vi "Solar Position Calculator - Meeus.vi"(11 "Observer's Latitude":dbl=39.977726 format="%#_8g", 13 "Observer's Longitude":dbl=105.274512 format="%#_9g") -> (9 "LST [Deg]":ext=222.68484852563896581 format="%_6g", 14 "Apparent Solar RA (deg)":dbl=243.2050632762713 format="%.6f", 15 "Apparent Solar Dec (deg)":dbl=-21.152223700920082 format="%.6f", 16 "Solar Altitude":dbl=25.94308858867875 format="%#_10g", 17 "Solar Azimuth":dbl=158.68124009009193 format="%#_10g", 18 "System Time and Date":T2={"current local time"=timestamp(3531489986.983003 s since 1904-01-01), "Julian Date"=2457354.2267004647, "LST [hh:mm:ss]"="14:50:44.4"} {"Julian Date" format="%_12f"}, 19 "Solar Position":T1={"Azimuth"=158.68124009009193, "Altitude wrt Horizon"=25.94308858867875, "Apparent RA (h:m:s)"="16:12:49.2", "Apparent Declination [dms]"="-21:9:8.005"} {"Altitude wrt Horizon" format="%.3f"; "Azimuth" format="%.3f"})   [LabVIEW 2015]
doc: "Solar Coordinates with High Accuracy, \"Astronomical Algorithms\" by Jean Meeus, pg. 166\n\nUsing data from Appendix III, (for the earth), calculate the earth's heliocentric longitude \"L\" and latitutde \"B\", and the radius vector \"R\" for a given instant as explained in chapter 32\n\nTime 'tau' is measured from JDE 2451545.0 in Julian mellenia (365250 days), NOT in centures and that the final values for \"L\" and \"B\" are in radians.\n\nChapter 32: \"Positions of the Planets\" \n The osculating orbit (using long series of periodic terms) is the \"instantaneous\" orbit with the following values:\n\n a = semi-major axis of the orbit\n lambda = mean longitude of the planet\n h = e sin (pi)\n k = e cos (pi)\n p = sin (1/2 i) sin (Omega)\n q = sin(1/2 i) cos (Omega)\n\n where 'e' is the orbital eccentricity\n 'pi' is the longitude of the perihelion\n 'i' is the inclination and\n 'Omega' is the longitude of the ascending node"
panel:
  out "Sun's Apparent Longitude\nCorrected for Aberration":dbl=245.13904264450866 format="%#_8g"
  out "Julian centuries (T)":ext=0.15904795894496178561 format="%_10g"
  out "Sun's Apparent Longitude":string="245:8:18.627"
  out "Sun's Apparent Longitude\nCorrected for Nutation and Aberration":dbl=245.13850753497218 format="%_8g"
  out "Equation \n25.10":dbl=-20.76572876500679
  out "Laskar True Obliquity [Deg]":dbl=23.43451957510621 format="%#_10g"
  out "Ecliptic Latitude [dms]":string="359:59:59.442"
  out "Ecliptic Latitude (FK)":dbl=359.9998448896821
  out "FK5 Longitude":dbl=245.14481090249893 format="%#_9g"
  out "Geocentric Solar Latitude":string="359:59:59.398"
  out "Deg:Min:Sec":string="245:8:41.319"
  out "series sum for d(epsilon) [\"]":dbl=-9.732610111354601 format="%#_4g"
  out "series sum for d(psi) [\"]":dbl=-1.9263943312994156 format="%#_5g"
  out "Laskar True Obliquity [DMS]":string="23:26:4.270"
  out "Latitude Correction \nfor Change from VSOP to FK5 System\n[arc seconds]":dbl=0.043620587030384496 format="%#_2g"
  in  "Longitude Correction\nfor Change from VSOP to FK6 System\n[deg] see page 166-169 of Meeus":dbl=-2.5e-05 format="%_4f"
  out "L' [FK5 System]":dbl=244.9226380620143 format="%#_5g"
  out "T":dbl=0.15904795894496176 format="%#_10g"
  out "Geocentric Latitude of the Sun [deg]":dbl=359.99983277285236 format="%#_4g"
  out "Geocentric Longitude of the Sun":dbl=245.14483590249893 format="%#_9g"
  out "B [deg]":dbl=0.00016722714764220623 format="%#_4g"
  out "L [0-360]":dbl=65.14483590249893 format="%#_8g"
  out "L [deg]":dbl=5825.144835902499 format="%#_10g"
  out "R [AU]":dbl=0.9867123004384141 format="%#_8g"
  out "B [rad]":dbl=2.918664325075171e-06 format="%#_3f"
  out "L [rad]":dbl=101.66795679204338 format="%#_10g"
  out "Julian Millenia (tau)":dbl=0.015904795894496178 format="%#_10g"
  in  "L0 - Earthm [64 terms]":dbl[][](array[numeric])=[[175347046.0, 0.0, 0.0], [3341656.0, 4.6692568, 6283.07585], [34894.0, 4.6261, 12566.1517], [3497.0, 2.7441, 5753.3849], [3418.0, 2.8289, 3.5231], [3136.0, 3.6277, 77713.7715], [2676.0, 4.4181, 7860.4194], [2343.0, 6.1352, 3930.2097], [1324.0, 0.7425, 11506.7698], [1273.0, 2.0371, 529.691], [1199.0, 1.1096, 1577.3435], [990.0, 5.233, 5884.927], [902.0, 2.045, 26.298], [857.0, 3.508, 398.149], [780.0, 1.179, 5223.694], [753.0, 2.533, 5507.553], [505.0, 4.583, 18849.228], [492.0, 4.205, 775.523], [357.0, 2.92, 0.067], [317.0, 5.849, 11790.629], [284.0, 1.899, 796.298], [271.0, 0.315, 10977.079], [243.0, 0.345, 5486.778], [206.0, 4.806, 2544.314], [205.0, 1.869, 5573.143], [202.0, 2.458, 6069.777], [156.0, 0.833, 213.299], [132.0, 3.411, 2942.463], [126.0, 1.083, 20.775], [115.0, 0.645, 0.98], [103.0, 0.636, 4694.003], [102.0, 0.976, 15720.839], [102.0, 4.267, 7.114], [99.0, 6.21, 2146.17], [98.0, 0.68, 155.42], [86.0, 5.98, 161000.69], [85.0, 1.3, 6275.96], [85.0, 3.67, 71430.7], [80.0, 1.81, 17260.15], [79.0, 3.04, 12036.46], [75.0, 1.76, 5088.63], [74.0, 3.5, 3154.69], [74.0, 4.68, 801.82], [70.0, 0.83, 9437.76], [62.0, 3.98, 8827.39], [61.0, 1.82, 7084.9], [57.0, 2.78, 6286.6], [56.0, 4.39, 14143.5], [56.0, 3.47, 6279.55], [52.0, 0.19, 12139.55], [52.0, 1.33, 1748.02], [51.0, 0.28, 5856.48], [49.0, 0.49, 1194.45], [41.0, 5.37, 8429.24], [41.0, 2.4, 19651.05], [39.0, 6.17, 10447.39], [37.0, 6.04, 10213.29], [37.0, 2.57, 1059.38], [36.0, 1.71, 2352.87], [36.0, 1.78, 6812.77], [33.0, 0.59, 17789.85], [30.0, 0.44, 83996.85], [30.0, 2.74, 1349.87], [25.0, 3.16, 4690.48]] format="%#_12g"
  in  "L1 - Earth [34 terms]":dbl[][](array[numeric])=[[628331966747.0, 0.0, 0.0], [206059.0, 2.678235, 6283.07585], [4303.0, 2.678235, 12566.1517], [425.0, 1.59, 3.523], [119.0, 5.796, 26.298], [109.0, 2.966, 1577.344], [93.0, 2.59, 18849.23], [72.0, 1.14, 529.69], [68.0, 1.87, 398.15], [67.0, 4.41, 5507.55], [59.0, 2.89, 5223.69], [56.0, 2.17, 155.42], [45.0, 0.4, 796.3], [36.0, 0.47, 775.52], [29.0, 2.65, 7.11], [21.0, 5.34, 0.98], [19.0, 1.85, 5486.78], [19.0, 4.97, 213.3], [17.0, 2.99, 6275.96], [16.0, 0.03, 2544.31], [16.0, 1.43, 2146.17], [15.0, 1.21, 10977.08], [12.0, 2.83, 1748.02], [12.0, 3.26, 5088.63], [12.0, 5.27, 1194.45], [12.0, 2.08, 4694.0], [11.0, 0.77, 553.57], [10.0, 1.3, 6286.6], [10.0, 4.24, 1349.87], [9.0, 2.7, 242.73], [9.0, 5.64, 951.72], [8.0, 5.3, 2352.87], [6.0, 2.65, 9437.76], [6.0, 4.67, 4690.48]] format="%#_12g"
  in  "L2 - Earth [20 terms]":dbl[][](array[numeric])=[[52919.0, 0.0, 0.0], [8720.0, 1.0721, 6283.0758], [309.0, 0.867, 12566.152], [27.0, 0.05, 3.52], [16.0, 5.19, 26.3], [16.0, 3.68, 155.42], [10.0, 0.76, 18849.23], [9.0, 2.06, 77713.77], [7.0, 0.83, 775.52], [5.0, 4.66, 1577.34], [4.0, 1.03, 7.11], [4.0, 3.44, 5573.14], [3.0, 5.14, 796.3], [3.0, 6.05, 5507.55], [3.0, 1.19, 242.73], [3.0, 6.12, 529.69], [3.0, 0.31, 398.15], [3.0, 2.28, 553.57], [2.0, 4.38, 5223.69], [2.0, 3.75, 0.98]] format="%#_12g"
  in  "L3 - Earth [7 terms]":dbl[][](array[numeric])=[[289.0, 5.844, 6283.076], [35.0, 0.0, 0.0], [17.0, 5.49, 12566.15], [3.0, 5.2, 155.42], [1.0, 4.72, 3.52], [1.0, 5.3, 18849.23], [1.0, 5.97, 242.73]] format="%#_12g"
  in  "L4 - Earth [3 terms]":dbl[][](array[numeric])=[[114.0, 3.142, 0.0], [8.0, 4.13, 6283.08], [1.0, 3.84, 12566.15]] format="%#_12g"
  in  "L5 - Earth [1 term]":dbl[][](array[numeric])=[[1.0, 3.14, 0.0]] format="%#_12g"
  in  "R0 - Earth [40 terms]":dbl[][](array[numeric])=[[100013989.0, 0.0, 0.0], [1670700.0, 3.0984635, 6283.07585], [13956.0, 3.05525, 12566.1517], [3084.0, 5.1985, 77713.7715], [1628.0, 1.1739, 5753.5849], [1576.0, 2.8469, 7860.4194], [925.0, 5.453, 11506.77], [542.0, 4.564, 3930.21], [472.0, 3.661, 5884.927], [346.0, 0.964, 5507.553], [329.0, 5.9, 5223.694], [307.0, 0.299, 5573.143], [243.0, 4.273, 11790.629], [212.0, 5.847, 1577.344], [186.0, 5.022, 10977.079], [175.0, 3.012, 18849.228], [110.0, 5.055, 5486.778], [98.0, 0.89, 6069.78], [86.0, 5.69, 15720.84], [86.0, 1.27, 161000.69], [65.0, 0.27, 17260.15], [63.0, 0.92, 529.69], [57.0, 2.01, 83996.85], [56.0, 5.24, 71430.7], [49.0, 3.25, 2544.31], [47.0, 2.58, 775.52], [45.0, 5.54, 9437.76], [43.0, 6.01, 6275.96], [39.0, 5.36, 4694.0], [38.0, 2.39, 8827.39], [37.0, 0.83, 19651.05], [37.0, 4.9, 12139.55], [36.0, 1.67, 12036.46], [35.0, 1.84, 2942.46], [33.0, 0.24, 7084.9], [32.0, 0.18, 5088.63], [32.0, 1.78, 398.15], [28.0, 1.21, 6286.6], [28.0, 1.9, 6279.55], [26.0, 4.59, 10447.39]] format="%#_12g"
  in  "R1 - Earth [10 terms]":dbl[][](array[numeric])=[[103019.0, 1.10749, 6283.07585], [1721.0, 1.0644, 12566.1517], [702.0, 3.142, 0.0], [32.0, 1.02, 18849.23], [31.0, 2.84, 5507.55], [25.0, 1.32, 5223.69], [18.0, 1.42, 1577.34], [10.0, 5.91, 10977.08], [9.0, 1.42, 6275.96], [9.0, 0.27, 5486.78]] format="%#_12g"
  in  "R2 - Earth [6-terms]":dbl[][](array[numeric])=[[4359.0, 5.7846, 6283.07585], [124.0, 5.579, 12566.152], [12.0, 3.14, 0.0], [9.0, 3.63, 77713.77], [6.0, 1.87, 5573.14], [3.0, 5.47, 18849.23]] format="%#_12g"
  in  "R4 - Earth [1-term]":dbl[][](array[numeric])=[[4.0, 2.56, 6283.08]] format="%#_12g"
  in  "R3 - Earth [2-terms]":dbl[][](array[numeric])=[[145.0, 4.273, 6283.076], [7.0, 3.92, 12566.15]] format="%#_12g"
  in  "B1 - Earth [2 terms]":dbl[][](array[numeric])=[[9.0, 3.9, 5507.55], [6.0, 1.73, 5223.69]] format="%#_12g"
  in  "B0 - Earth [5 terms]":dbl[][](array[numeric])=[[280.0, 3.199, 84334.662], [102.0, 5.422, 5507.553], [80.0, 3.88, 5223.69], [44.0, 3.7, 2352.87], [32.0, 4.0, 1577.34]] format="%#_12g"
  # "These are the heliocentric longitude \"L\", latitude \"B\" \nreferred to the mean dynamical ecliptic."
  # "These are the geocentric \"L\" and \"B\"\nof the SUN, still referred to the mean\ndynamical ecliptic"
  # "The sun's longitude thus far is the true \n\"geometric\" longitude.  To obtain the apparent \nlongitude, lambda, the effects of nutation \nand abberation should be taken into account.\n\nNutation is calculated by means from Chapter 22."
  # "Converting to FK5 System"
  # "`"
  # "These corrections may be neglected\nwhen using the abridged VSOP version\nfrom Appendix III of Meeus"
  # "Using latlong.net, I determined the position of the Mesa Lab Dome to be\n39.977726, -105.274512"
  # "NOAA Solar Position Calculator \nNew: http://www.esrl.noaa.gov/gmd/grad/solcalc/\nOld http://www.srrb.noaa.gov/highlights/sunrise/azel.html\n\nDefault Values for Mesa Lab Spar\n39.977727 degrees latitude\n-105.274512 degrees (west of prime meridian)\n\nJPL Horizons Calculator \nhttp://ssd.jpl.nasa.gov/horizons.cgi\n\nEphemeris Type: Observer\nTarget Body: Sun [Sol] \nObserver Location: user defined (105N15'39.6\"E, 39:59:27.6\" N, 6000 ft)\nTime Span: user defined Start: 2015-03-24, Stop 2015-03-25, Step - 1min)\nTable Settings: Qantities 2,13,36, CSV format = YES, angle format can be either DEG or HMS\nDisplay/Output: default (can be sent to a text file)"
  # "Ecliptic Solar Coordinates"
  # "Horizon Solar Coordinates"
  # "Apparent Equatorial Solar Coordinates"
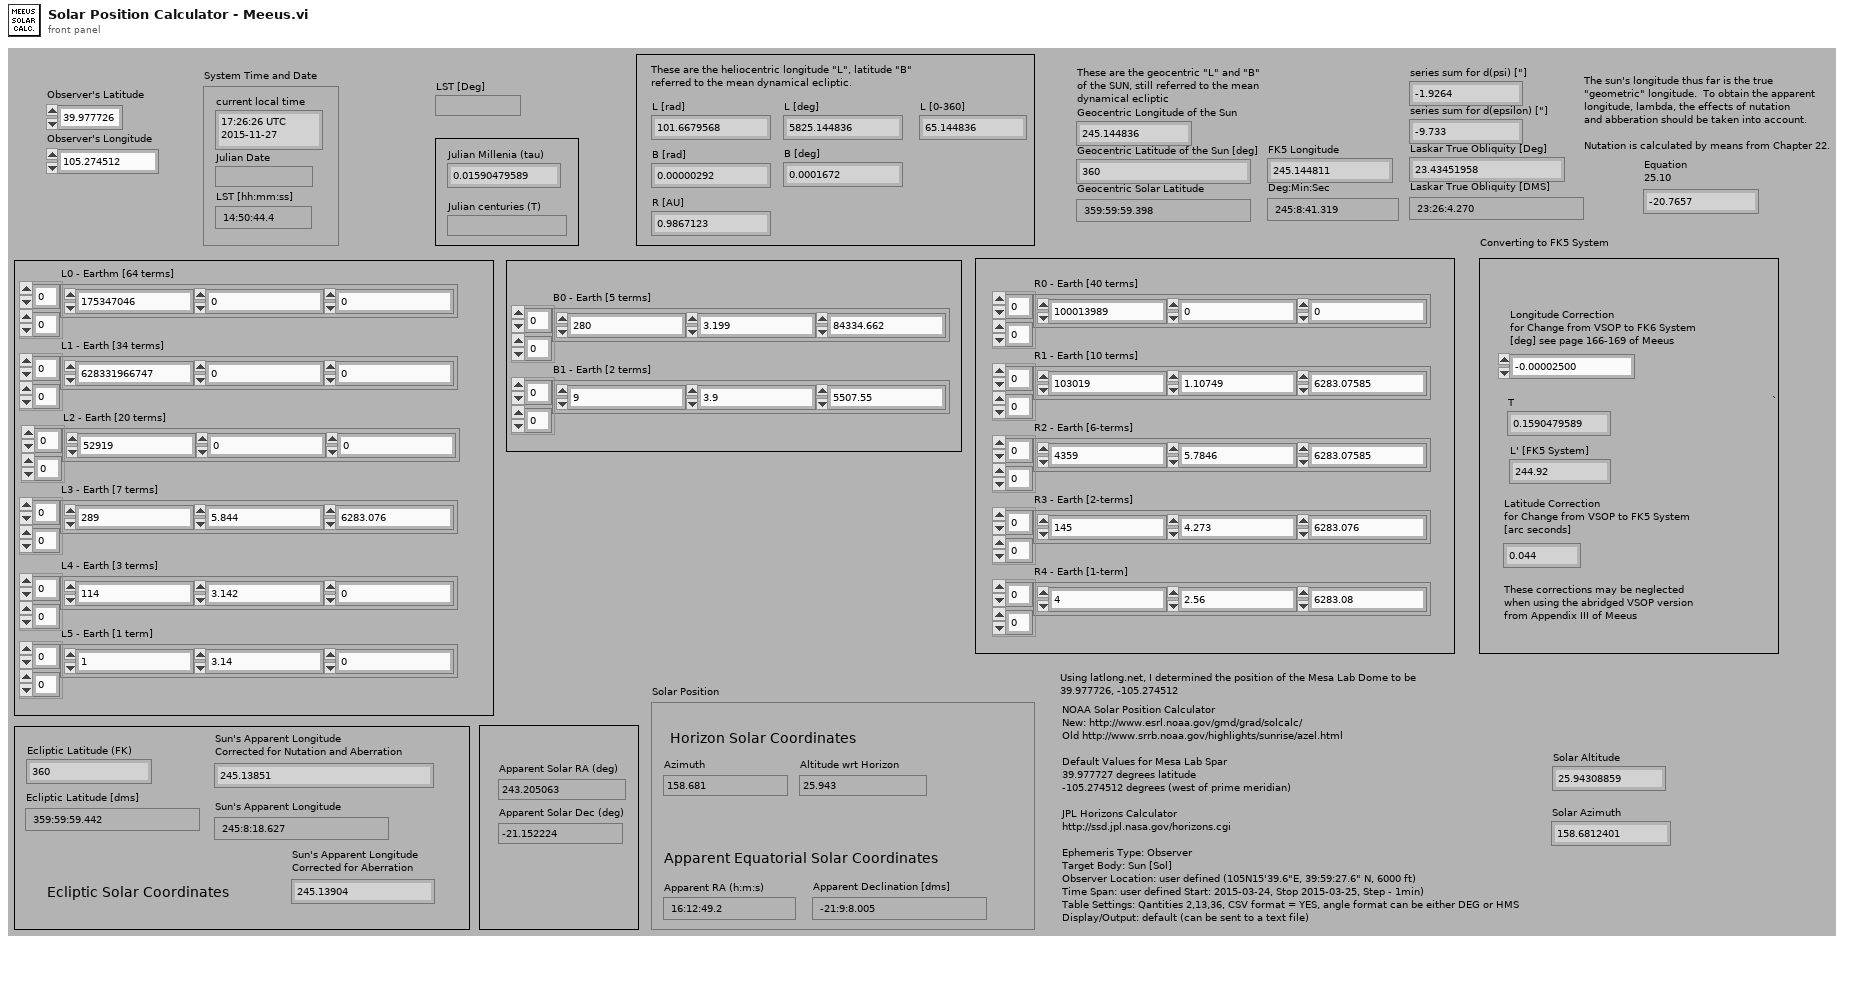
[diagram p1: front panel]
types:
  T1 = cluster{"Azimuth":dbl, "Altitude wrt Horizon":dbl, "Apparent RA (h:m:s)":string, "Apparent Declination [dms]":string}
  T2 = cluster{"current local time":timestamp, "Julian Date":ext, "LST [hh:mm:ss]":string}
  T3 = cluster{"current time":timestamp, "JD":ext, "LST [hh:mm:ss]":string}
  T4 = cluster{"Az":dbl, "Alt":dbl, "RA (h:m:s)":string, "Deg:Min:Sec":string}
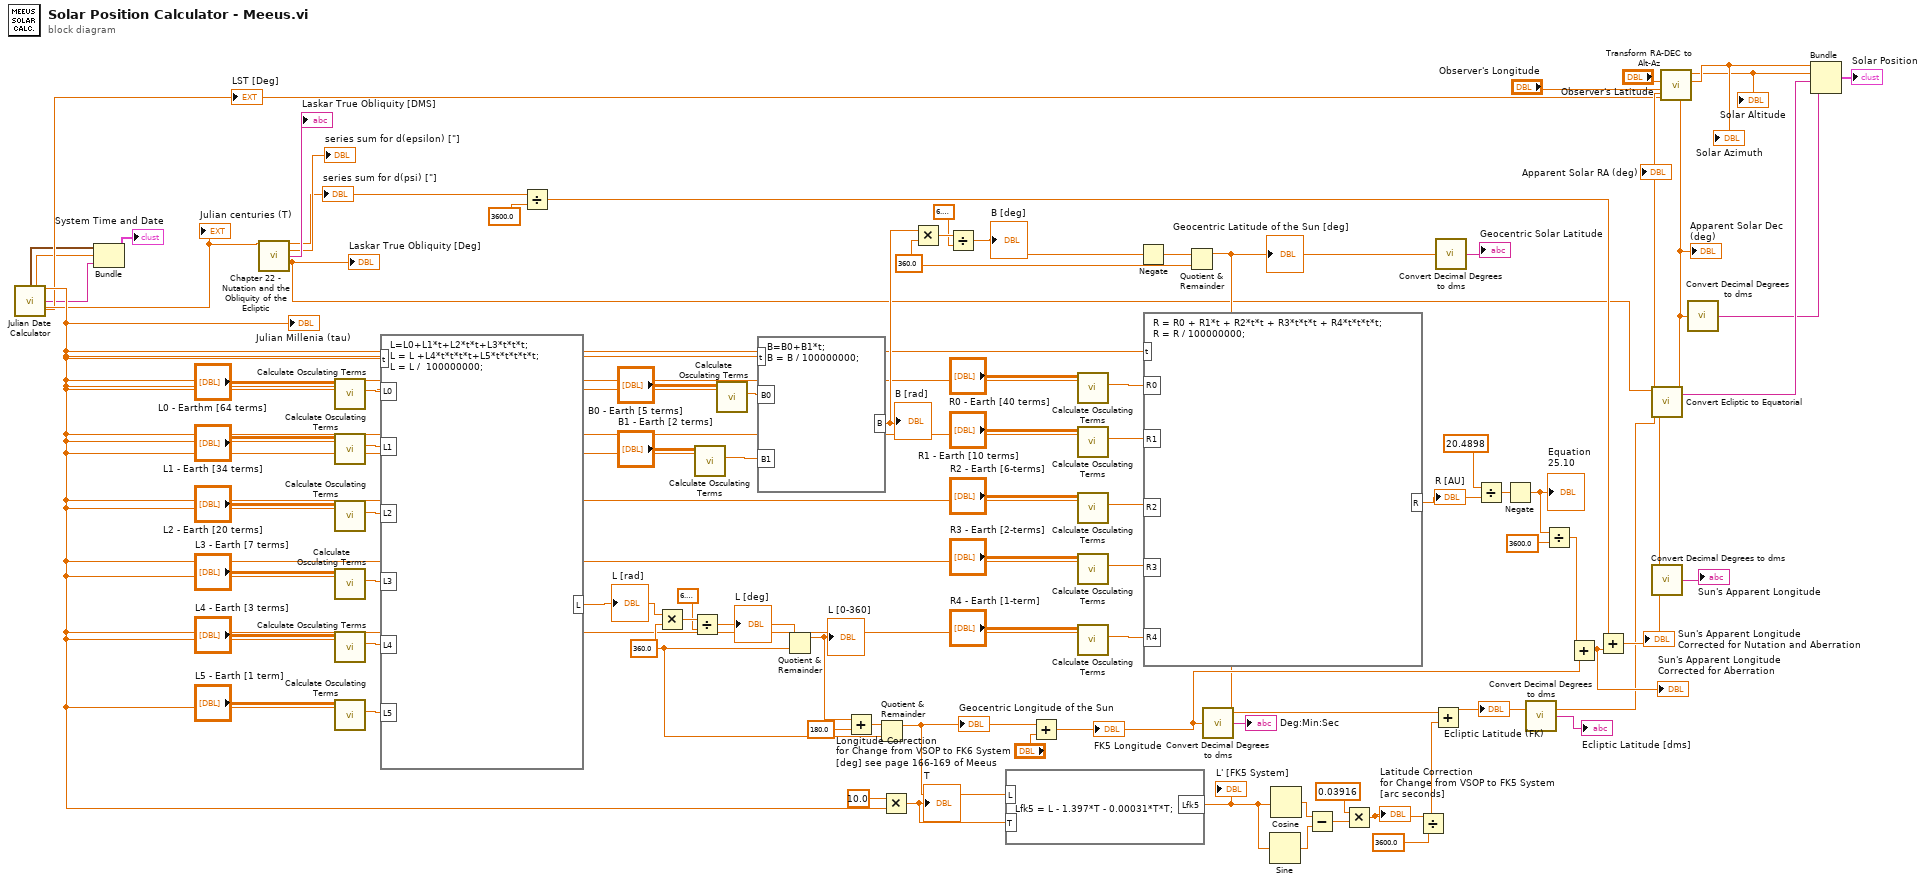
[diagram p0: block diagram]
diagram:
  w49 = 360.0 ("y")
  w53 = 360.0 ("y")
  n1 = call "Julian Date Calculator.vi"() -> ("current time"=w1:timestamp, "JD"=w4:ext, "tau (measured in Julian millenia)"=w12:dbl, "LST [hh:mm:ss]"=w2:string, "T (measured in Julian centuries)"=w11:ext, "LST [Deg]"=w10:ext)  [unwired: 3 in, 7 out]
  "Julian Millenia (tau)" <- w12
  "LST [Deg]" <- w10
  "Julian centuries (T)" <- w11
  n2 = Bundle("current time"=w1, "JD"=w4, "LST [hh:mm:ss]"=w2) -> (→"System Time and Date":T3)  [unwired: 1 in]
  n3 = call "Chapter 22 - Nutation and the Obliquity of the Ecliptic.vi"("T"=w11) -> ("series sum for d(psi) [\"]"=w27:dbl, "series sum for d(epsilon) [\"]"=→"series sum for d(epsilon) [\"]":dbl, "Laskar True Obliquity [DMS]"=→"Laskar True Obliquity [DMS]":string, "Laskar True Obliquity [Deg]"=w17:dbl)  [unwired: 11 out]
  "series sum for d(psi) [\"]" <- w27
  "Laskar True Obliquity [Deg]" <- w17
  n4 = call "Calculate Osculating Terms.vi"("tau"=w12, "ABC Coefficient Array"="L0 - Earthm [64 terms]") -> ("Series Sum"=w69:dbl)  [unwired: 9 out]
  n5 = call "Calculate Osculating Terms.vi"("tau"=w12, "ABC Coefficient Array"="L1 - Earth [34 terms]") -> ("Series Sum"=w68:dbl)  [unwired: 9 out]
  n6 = call "Calculate Osculating Terms.vi"("tau"=w12, "ABC Coefficient Array"="L2 - Earth [20 terms]") -> ("Series Sum"=w67:dbl)  [unwired: 9 out]
  n7 = call "Calculate Osculating Terms.vi"("tau"=w12, "ABC Coefficient Array"="L3 - Earth [7 terms]") -> ("Series Sum"=w66:dbl)  [unwired: 9 out]
  n8 = call "Calculate Osculating Terms.vi"("tau"=w12, "ABC Coefficient Array"="L4 - Earth [3 terms]") -> ("Series Sum"=w65:dbl)  [unwired: 9 out]
  n9 = call "Calculate Osculating Terms.vi"("tau"=w12, "ABC Coefficient Array"="L5 - Earth [1 term]") -> ("Series Sum"=w64:dbl)  [unwired: 9 out]
  n10 = formula code="L=L0+L1*t+L2*t*t+L3*t*t*t;\nL = L +L4*t*t*t*t+L5*t*t*t*t*t;\nL = L /  100000000;"("L0"=w69, "L1"=w68, "L2"=w67, "L3"=w66, "L4"=w65, "L5"=w64, "t"=w12) -> ("L"=w63:dbl)
  "L [rad]" <- w63
  n11 = Divide(x=w27, y=3600.0) -> (x/y=w26:dbl)
  n12 = Multiply(x=w63, y=w53) -> (x*y=w62:dbl)
  n13 = Divide(x=w62, y=6.283185307179586) -> (x/y=w60:dbl)
  "L [deg]" <- w60
  n14 = call "Calculate Osculating Terms.vi"("tau"=w12, "ABC Coefficient Array"="B1 - Earth [2 terms]") -> ("Series Sum"=w70:dbl)  [unwired: 9 out]
  n15 = call "Calculate Osculating Terms.vi"("tau"=w12, "ABC Coefficient Array"="B0 - Earth [5 terms]") -> ("Series Sum"=w71:dbl)  [unwired: 9 out]
  n16 = formula code="B=B0+B1*t;\nB = B / 100000000;"("B0"=w71, "B1"=w70, "t"=w12) -> ("B"=w57:dbl)
  "B [rad]" <- w57
  n17 = Quotient & Remainder(x=w60, y=w53) -> (x-y*floor(x/y)=w56:dbl)  [unwired: 1 out]
  "L [0-360]" <- w56
  n18 = Add(x=w56, y=180.0) -> (x+y=w54:dbl)
  n19 = Quotient & Remainder(x=w54, y=w53) -> (x-y*floor(x/y)=w37:dbl)  [unwired: 1 out]
  "Geocentric Longitude of the Sun" <- w37
  n20 = Multiply(x=10.0, y=w12) -> (x*y=w51:dbl)
  "T" <- w51
  n21 = Multiply(x=w57, y=w49) -> (x*y=w59:dbl)
  n22 = Divide(x=w59, y=6.283185307179586) -> (x/y=w48:dbl)
  "B [deg]" <- w48
  n23 = formula code="Lfk5 = L - 1.397*T - 0.00031*T*T;"("T"=w51, "L"=w37) -> ("Lfk5"=w46:dbl)
  "L' [FK5 System]" <- w46
  n24 = Add(x=w37, y="Longitude Correction\nfor Change from VSOP to FK6 System\n[deg] see page 166-169 of Meeus") -> (x+y=w29:dbl)
  "FK5 Longitude" <- w29
  n25 = call "Calculate Osculating Terms.vi"("tau"=w12, "ABC Coefficient Array"="R0 - Earth [40 terms]") -> ("Series Sum"=w76:dbl)  [unwired: 9 out]
  n26 = call "Calculate Osculating Terms.vi"("tau"=w12, "ABC Coefficient Array"="R1 - Earth [10 terms]") -> ("Series Sum"=w75:dbl)  [unwired: 9 out]
  n27 = call "Calculate Osculating Terms.vi"("tau"=w12, "ABC Coefficient Array"="R2 - Earth [6-terms]") -> ("Series Sum"=w74:dbl)  [unwired: 9 out]
  n28 = call "Calculate Osculating Terms.vi"("tau"=w12, "ABC Coefficient Array"="R3 - Earth [2-terms]") -> ("Series Sum"=w73:dbl)  [unwired: 9 out]
  n29 = call "Calculate Osculating Terms.vi"("tau"=w12, "ABC Coefficient Array"="R4 - Earth [1-term]") -> ("Series Sum"=w72:dbl)  [unwired: 9 out]
  n30 = Negate(x=w48) -> (-x=w50:dbl)
  n31 = formula code="R = R0 + R1*t + R2*t*t + R3*t*t*t + R4*t*t*t*t;\nR = R / 100000000;"("R0"=w76, "R1"=w75, "R2"=w74, "R3"=w73, "R4"=w72, "t"=w12) -> ("R"=w32:dbl)
  "R [AU]" <- w32
  n32 = Quotient & Remainder(x=w50, y=w49) -> (x-y*floor(x/y)=w20:dbl)  [unwired: 1 out]
  "Geocentric Latitude of the Sun [deg]" <- w20
  n33 = call "Convert Decimal Degrees to dms.vi"("Decimal Degrees"=w29) -> ("Deg:Min:Sec"=→"Deg:Min:Sec":string)
  n34 = Sine(x=w46) -> (sin(x)=w45:dbl)
  n35 = Cosine(x=w46) -> (cos(x)=w47:dbl)
  n36 = Subtract(x=w47, y=w45) -> (x-y=w44:dbl)
  n37 = Multiply(x=0.03916 ("x-y"), y=w44) -> (x*y=w36:dbl)
  "Latitude Correction \nfor Change from VSOP to FK5 System\n[arc seconds]" <- w36
  n38 = Divide(x=w36, y=3600.0) -> (x/y=w34:dbl)
  n39 = Add(x=w20, y=w34) -> (x+y=w18:dbl)
  "Ecliptic Latitude (FK)" <- w18
  n40 = call "Convert Decimal Degrees to dms.vi"("Decimal Degrees"=w20) -> ("Deg:Min:Sec"=→"Geocentric Solar Latitude":string)
  n41 = Divide(x=20.4898, y=w32) -> (x/y=w30:dbl)
  n42 = Negate(x=w30) -> (-x=w23:dbl)
  "Equation \n25.10" <- w23
  n43 = call "Convert Decimal Degrees to dms.vi"("Decimal Degrees"=w18) -> ("Deg:Min:Sec"=→"Ecliptic Latitude [dms]":string)
  n44 = Divide(x=w23, y=3600.0) -> (x/y=w22:dbl)
  n45 = Add(x=w22, y=w29) -> (x+y=w25:dbl)
  "Sun's Apparent Longitude\nCorrected for Aberration" <- w25
  n46 = Add(x=w26, y=w25) -> (x+y=w19:dbl)
  "Sun's Apparent Longitude\nCorrected for Nutation and Aberration" <- w19
  n47 = call "Convert Ecliptic to Equatorial.vi"("Epsilon"=w17, "Lambda"=w19, "Beta"=w18) -> ("RA (h:m:s)"=w6:string, "Right Ascension (alpha) in degrees"=w16:dbl, "Declination (delta) in degrees"=w15:dbl)  [unwired: 4 out]
  "Apparent Solar RA (deg)" <- w16
  "Apparent Solar Dec (deg)" <- w15
  n48 = call "Convert Decimal Degrees to dms.vi"("Decimal Degrees"=w19) -> ("Deg:Min:Sec"=→"Sun's Apparent Longitude":string)
  n49 = call "Transform RA-DEC to Alt-Az.vi"("dec"=w15, "RA"=w16, "LST [Deg]"=w10, "Observer's Longitude"="Observer's Longitude", "Observer's Latitude (phi)"="Observer's Latitude") -> ("Az"=w8:dbl, "Alt"=w7:dbl)  [unwired: 1 in, 4 out]
  "Solar Azimuth" <- w8
  "Solar Altitude" <- w7
  n50 = call "Convert Decimal Degrees to dms.vi"("Decimal Degrees"=w15) -> ("Deg:Min:Sec"=w5:string)
  n51 = Bundle("Az"=w8, "Alt"=w7, "RA (h:m:s)"=w6, "Deg:Min:Sec"=w5) -> (→"Solar Position":T4)  [unwired: 1 in]
